vi "CleanUp.vi"(0 "object in":refnum<class "NewTestSkill.lvclass">, 5 "error in (no error)":errorcluster) -> (14 "object out":refnum<class "NewTestSkill.lvclass">, 19 "error out":errorcluster)   [LabVIEW 2022 SP3, in "NewTestSkill.lvclass"]
uses:
  NewTestSkill.lvclass
  Skill_class/Skill.lvclass
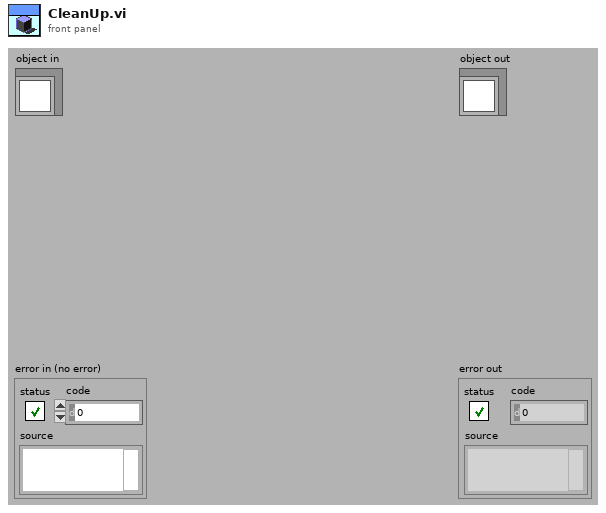
[diagram p1: front panel]
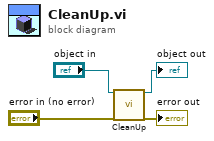
[diagram p0: block diagram]
diagram:
  n1 = call-parent "CleanUp.vi"("object in"="object in", "error in (no error)"="error in (no error)") -> ("object out"=→"object out":refnum<class "NewTestSkill.lvclass">, "error out"=→"error out":errorcluster)  [unwired: 16 in]
